vi "Test harness - Compare 2 Icons.vi"(7 "Type of file to test":T1=".vi", 9 "Debug":bool, 10 "Temp file location":T2=7 items=["User Home"=0, "User Desktop"=1, "User Documents"=2, "User Application Data"=3, "User Preferences"=4, "User Temporary"=5, "Public Documents"=6, "Public Application Data"=7, "Public Preferences"=8, "Public Cache"=13, "System Core Libraries"=9, "System Installed Libraries"=10, "Application Files"=11, "Boot Volume Root"=12], 11 "Application reference":refnum<vi>) -> (0 "error out":errorcluster, 2 "Cycle time (For debug)":dbl, 3 "Pass":bool)   [LabVIEW 2021]
uses:
  <vilib>/Utility/sysdir.llb/System Directory Type.ctl
  85a5cb5c-572b-4d5b-8973-222a2b0d8f2b.vi
  Test harness file type.ctl
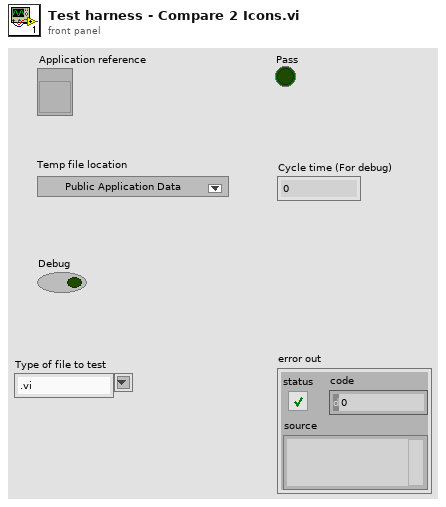
[diagram p1: front panel]
types:
  T1 = typedef "Test harness file type.ctl" = string
  T2 = typedef "System Directory Type.ctl" = i32
  T3 = typedef "imagedata.ctl" = cluster{"image type":i32, "image depth":i32, "image":u8[], "mask":u8[], "colors":u32[], "Rectangle":cluster{"left":i16, "top":i16, "right":i16, "bottom":i16}}
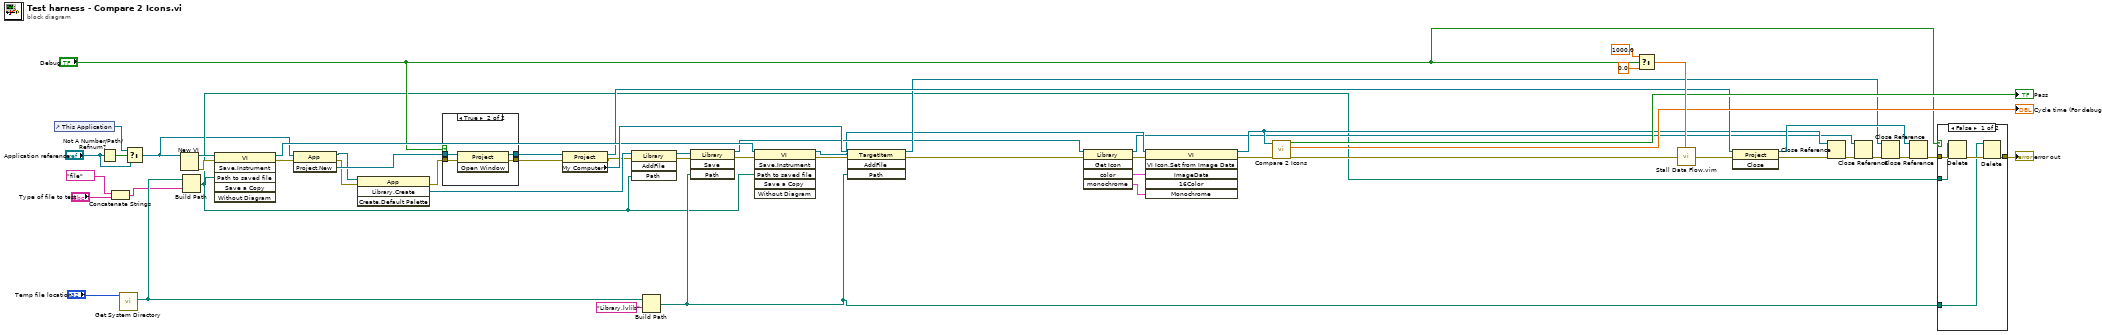
[diagram p0: block diagram]
diagram:
  n1 = control-ref of="This Application"() -> (w10:refnum<vi>)
  n2 = Not A Number/Path/Refnum?(number/path/refnum="Application reference") -> (NaN/Path/Refnum?=w11:bool)
  n3 = Concatenate Strings("file", "Type of file to test") -> (w1:string)
  n4 = call <vilib>:"Get System Directory.vi"("system directory type"="Temp file location") -> ("system directory"=w50:path)  [unwired: 10 in]
  n5 = Select(t=w10, s=w11, f="Application reference") -> (s? t:f=w9:refnum<vi>)
  n6 = New VI(11:w9) -> (0:w13:errorcluster, 3:w39:refnum<vi>)  [unwired: 1 in, 5 out]
  n7 = Build Path(base path=w50, name or relative path=w1) -> (appended path=w12:path)
  n8 = invoke class="VI" method="Save.Instrument"(reference=w39, error in=w13, "Path to saved file"=w12) -> (reference out=w34:refnum<vi>, error out=w38:errorcluster)  [unwired: 3 in, 4 out]
  n9 = invoke class="App" method="Project.New"(reference=w9, error in=w38) -> (reference out=w49:refnum<vi>, error out=w48:errorcluster, "Project:New"=w54:refnum<vi>)  [unwired: 1 in]
  n10 = invoke class="App" method="Library.Create"(reference=w49, error in=w48) -> (error out=w47:errorcluster, "Create Library"=w46:refnum<vi>)  [unwired: 2 in, 2 out]
  n11 = case shown="True" "Debug" {
    tunnel: w54 -> [w56 w61]
    tunnel: [w57 w60] -> w53
    tunnel: [w56 w59] -> w52
    tunnel: w47 -> [w57 w58]
    frame False {
    }
    frame True {
      n12 = invoke class="Project" method="Open Window"(reference=w61, error in=w58) -> (reference out=w59:refnum<vi>, error out=w60:errorcluster)  [unwired: 1 in, 1 out]
    }
  }
  n13 = property class="Project"(reference=w52, error in=w53) -> (reference out=w24:refnum<vi>, error out=w37:errorcluster, "My Computer"=w43:refnum<vi>)
  n14 = invoke class="Library" method="AddFile"(reference=w46, error in=w37, "Path"=w12) -> (reference out=w44:refnum<vi>, error out=w45:errorcluster)  [unwired: 1 in, 2 out]
  n15 = Build Path(base path=w50, name or relative path="Library.lvlib") -> (appended path=w15:path)
  n16 = invoke class="Library" method="Save"(reference=w44, error in=w45, "Path"=w15) -> (reference out=w22:refnum<vi>, error out=w42:errorcluster)  [unwired: 1 in, 2 out]
  n17 = invoke class="VI" method="Save.Instrument"(reference=w34, error in=w42, "Path to saved file"=w12) -> (reference out=w20:refnum<vi>, error out=w41:errorcluster)  [unwired: 3 in, 4 out]
  n18 = invoke class="TargetItem" method="AddFile"(reference=w43, error in=w41, "Path"=w15) -> (reference out=w23:refnum<vi>, error out=w21:errorcluster)  [unwired: 1 in, 2 out]
  n19 = invoke class="Library" method="Get Icon"(reference=w22, error in=w21) -> (reference out=w18:refnum<vi>, error out=w7:errorcluster, "color"=w6:T3, "monochrome"=w5:T3)  [unwired: 3 in, 1 out]
  n20 = invoke class="VI" method="VI Icon.Set from Image Data"(reference=w20, error in=w7, "ImageData"=w6, "Monochrome"=w5) -> (reference out=w19:refnum<vi>, error out=w4:errorcluster)  [unwired: 2 in, 4 out]
  n21 = call "Compare 2 Icons.vi"("error in (no error)"=w4, "VI Reference"=w19) -> ("error out"=w25:errorcluster, "Cycle time (For debug)"=→"Cycle time (For debug)":dbl, "Match?"=→"Pass":bool)  [unwired: 7 in]
  n22 = Select(t=1000.0, s="Debug", f=0.0) -> (s? t:f=w28:dbl)
  n23 = call "Stall Data Flow.vim"("value in"=w25, "milliseconds to wait"=w28) -> ("value out"=w29:errorcluster)  [unwired: 1 out]
  n24 = invoke class="Project" method="Close"(reference=w24, error in=w29) -> (reference out=w32:refnum<vi>, error out=w33:errorcluster)  [unwired: 1 in, 1 out]
  n25 = Close Reference(reference=w19, error in (no error)=w33) -> (error out=w40:errorcluster)
  n26 = Close Reference(reference=w18, error in (no error)=w40) -> (error out=w36:errorcluster)
  n27 = Close Reference(reference=w23, error in (no error)=w36) -> (error out=w35:errorcluster)
  n28 = Close Reference(reference=w32, error in (no error)=w35) -> (error out=w17:errorcluster)
  n29 = case shown="False" "Debug" {
    tunnel: w17 -> [w66 w67]
    tunnel: [w64 w67] -> w16
    tunnel: w12 -> [w63 _]
    tunnel: w15 -> [w62 _]
    frame False {
      n30 = Delete(path (use dialog)=w63, error in=w66) -> (error out=w65:errorcluster)  [unwired: 3 in, 2 out]
      n31 = Delete(path (use dialog)=w62, error in=w65) -> (error out=w64:errorcluster)  [unwired: 3 in, 2 out]
    }
    frame True {
    }
  }
  "error out" <- w16
